vi "Step Type Selection UI.vi"() -> (2 "Cancelled":bool, 3 "Step Type":T1)   [LabVIEW 2018, in "Temp Recipe.lvlib" / "Recipe Editor.lvclass"]
uses:
  Recipe Editor.lvclass
  Step Type.ctl
panel:
  in  "Cancel Button":bool
  in  "OK Button":bool
  in  "Selection":T1
  # "Select step type to add:"
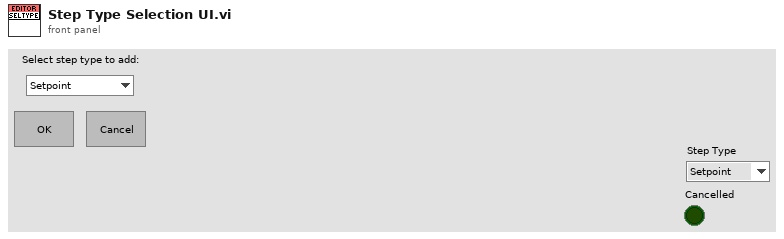
[diagram p1: front panel]
types:
  T1 = typedef "Temp Recipe.lvlib/Recipe Editor.lvclass/Step Type.ctl" = enum16{"Setpoint", "Step Rate", "Rate Duration", "Delay"}
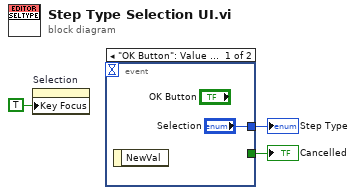
[diagram p0: block diagram]
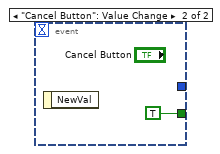
[diagram p2: hidden frame]
diagram:
  n1 = property on="Selection" class="Enum (strict)"("Key Focus"=TRUE) -> ()  [unwired: 2 in, 2 out]
  n2 = event shown="[0] \"OK Button\": Value Change" {
    selector: _ -> [_ _]
    dyn-events: _ -> [_ _]
    timeout: _ -> [_ _]
    tunnel: ["Selection" _] -> w3
    tunnel: [_ TRUE] -> w2
    event "OK Button": Value Change {
      n3 = event-data() -> ()  [unwired: 1 in, 1 out]
    }
    event "Cancel Button": Value Change {
      n4 = event-data() -> ()  [unwired: 1 in, 1 out]
    }
  }
  "Step Type" <- w3
  "Cancelled" <- w2
